vi "delete update counters.vi"(8 "This VI":refnum<vi>, 10 "just quit":bool) -> (0 "This VI":refnum<vi>)   [LabVIEW 2010]
uses:
  <vilib>/Utility/sysdir.llb/System Directory Type.ctl
panel:
  in  "Close":bool
  # "The update countdown counters were all deleted.\nRestart the GUIs to check for updates.\n\nThe Csv Convert will be closed."
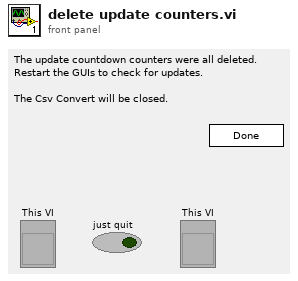
[diagram p1: front panel]
types:
  T1 = typedef "System Directory Type.ctl" = i32
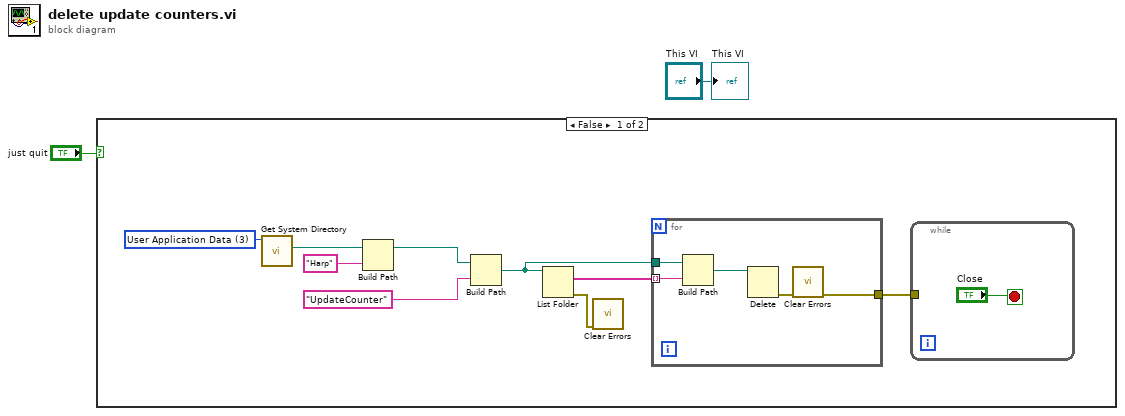
[diagram p0: block diagram]
diagram:
  n1 = case shown="False" "just quit" {
    frame False {
      w10 = T1 3 items=["User Home"=0, "User Desktop"=1, "User Documents"=2, "User Application Data"=3, "User Preferences"=4, "User Temporary"=5, "Public Documents"=6, "Public Application Data"=7, "Public Preferences"=8, "Public Cache"=13, "System Core Libraries"=9, "System Installed Libraries"=10, "Application Files"=11, "Boot Volume Root"=12] ("system directory type")
      n2 = call <vilib>:"Get System Directory.vi"("system directory type"=w10) -> ("system directory"=w9:path)  [unwired: 10 in]
      n3 = Build Path(base path=w9, name or relative path="Harp") -> (appended path=w8:path)
      n4 = Build Path(base path=w8, name or relative path="UpdateCounter") -> (appended path=w5:path)
      n5 = List Folder(path=w5) -> (filenames=w6:string[], error out=w4:errorcluster)  [unwired: 3 in, 2 out]
      n6 = call <vilib>:"Clear Errors.vi"("error in (no error)"=w4) -> ()  [unwired: 6 in, 1 out]
      n7 = for {
        tunnel: w6 -> [w17] mode=indexing
        tunnel: w5 -> [w16]
        tunnel: [w13] -> w3
        n8 = Build Path(base path=w16, name or relative path=w17) -> (appended path=w15:path)
        n9 = Delete(path (use dialog)=w15) -> (error out=w14:errorcluster)  [unwired: 4 in, 2 out]
        n10 = call <vilib>:"Clear Errors.vi"("error in (no error)"=w14) -> ("error out"=w13:errorcluster)  [unwired: 6 in]
      }
      n11 = while {
        tunnel: w3 -> [_]
        stop <- "Close" stop-if-true
      }
    }
    frame True {
    }
  }
  "This VI" <- "This VI"
